vi "disable_all.vi"(8 "error in (no error)":errorcluster caption="错误输入（无错误）", 11 "MotorSystem 输入":refnum<class "MotorSystem.lvclass">) -> (0 "error out":errorcluster caption="错误输出", 3 "MotorSystem 输出":refnum<class "MotorSystem.lvclass">)   [LabVIEW 2016, in "MotionControl.lvlib" / "MotorSystem.lvclass"]
uses:
  <userlib>/MotionControl/MotorSystem/MotorSystem.lvclass
  <userlib>/MotionControl/MotorSystem/MotorSystem.lvclass/MotorSystem.ctl
  <userlib>/MotionControl/OneMotion/OneMotion.lvclass/OneMotion.ctl
  <userlib>/MotionControl/OneMotion/OneMotion.lvclass
  <userlib>/UISimCanFunc_wrapper/UISimCanFunc_wrapper.lvlib
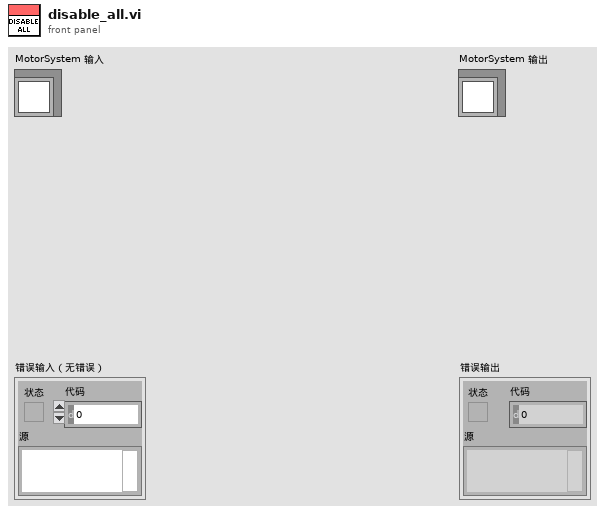
[diagram p1: front panel]
types:
  T1 = typedef "MotionControl.lvlib/MotorSystem.lvclass/MotionCluster.ctl" = cluster{"OneMotion.lvclass":refnum<class "OneMotion.lvclass">, "connected?":bool, "default enabled?":bool, "enabled?":bool}
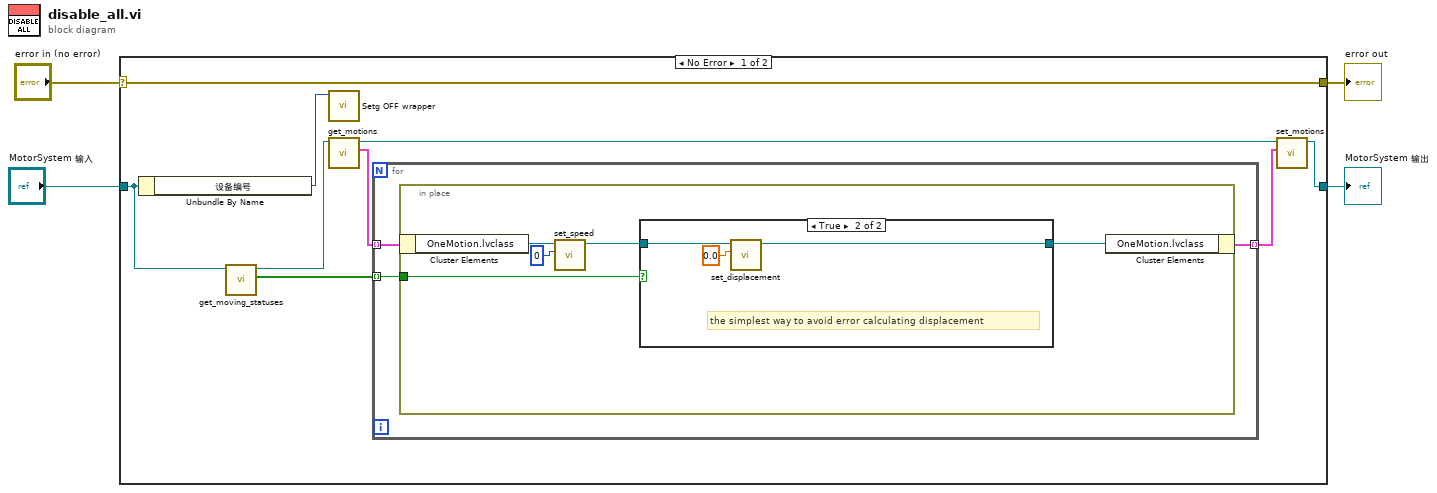
[diagram p0: block diagram]
diagram:
  n1 = case shown="No Error" "error in (no error)" {
    selector: "error in (no error)" -> [w13 w27]
    tunnel: [w13 w27] -> w3
    tunnel: [w8 w26] -> w1
    tunnel: "MotorSystem 输入" -> [w7 w26]
    frame No Error {
      n2 = Unbundle By Name(w7) -> ("设备编号"=w12:u32)
      n3 = call <userlib>:"get_moving_statuses.vi"("MotorSystem输入"=w7) -> ("moving?"=w5:bool[], "MotorSystem输出"=w6:refnum<class "MotorSystem.lvclass">)  [unwired: 8 in, 1 out]
      n4 = call <userlib>:"Setg OFF wrapper.vi"("dwDevIndex"=w12) -> ()  [unwired: 9 in, 2 out]
      n5 = call <userlib>:"get_motions.vi"("MotorSystem输入"=w6) -> ("motions"=w11:T1[], "MotorSystem输出"=w10:refnum<class "MotorSystem.lvclass">)  [unwired: 8 in, 1 out]
      n6 = for {
        tunnel: w11 -> [w16] mode=indexing
        tunnel: [w15] -> w9 mode=indexing
        tunnel: w5 -> [w14] mode=indexing
        n7 = in-place {
          in-place-border: w14 -> [w21]
          n8 = in-place-cluster #1(w16) -> ("OneMotion.lvclass"=w20:refnum<class "OneMotion.lvclass">)
          n9 = call-dynamic "set_speed.vi"("speed"=0, "OneMotion 输入"=w20) -> ("OneMotion 输出"=w18:refnum<class "OneMotion.lvclass">)  [unwired: 8 in, 1 out]
          n10 = case shown="True" w21 {
            tunnel: w18 -> [w22 w25]
            tunnel: [w22 w24] -> w17
            frame False {
            }
            frame True {
              # "the simplest way to avoid error calculating displacement"
              n11 = call <userlib>:"set_displacement.vi"("displacement"=0.0, "OneMotion输入"=w25) -> ("OneMotion输出"=w24:refnum<class "OneMotion.lvclass">)  [unwired: 8 in, 1 out]
            }
          }
          n12 = in-place-cluster #1("OneMotion.lvclass"=w17) -> (w15:T1)
        }
      }
      n13 = call <userlib>:"set_motions.vi"("motions"=w9, "MotorSystem输入"=w10) -> ("MotorSystem输出"=w8:refnum<class "MotorSystem.lvclass">)  [unwired: 8 in, 1 out]
    }
    frame Error {
    }
  }
  "error out" <- w3
  "MotorSystem 输出" <- w1
